vi "test Add Log File.vi"(8 "error in (no error)":errorcluster, 11 "TestCase in":refnum<class "Embedded Data Logger Scripting Unit Tests.lvclass">) -> (0 "error out":errorcluster, 3 "TestCase out":refnum<class "Embedded Data Logger Scripting Unit Tests.lvclass">)   [LabVIEW 2019, in "Embedded Data Logger Scripting Unit Tests.lvclass"]
uses:
  Embedded Data Logger Scripting Unit Tests.lvclass
  C:/Dev/GitHub/niveristand-custom-device-testing-tools/VeriStandScriptingTestCase/VeriStandScriptingTestCase.lvclass
  niveristand-custom-device-testing-tools/VeriStandScriptingTestCase/VeriStandScriptingTestCase.lvclass/VeriStandScriptingTestCase.ctl
  niveristand-custom-device-testing-tools/VeriStandScriptingTestCase/Read Target.vi
  NationalInstruments.VeriStand.SystemDefinitionAPI
  <vilib>/addons/_JKI Toolkits/VI Tester/TestCase.llb/TestCase.lvclass
  Embedded Data Logger Scripting.lvlib
  C:/Program Files (x86)/National Instruments/LabVIEW 2019/vi.lib/addons/_JKI Toolkits/VI Tester/TestCase.llb/TestCase.lvclass
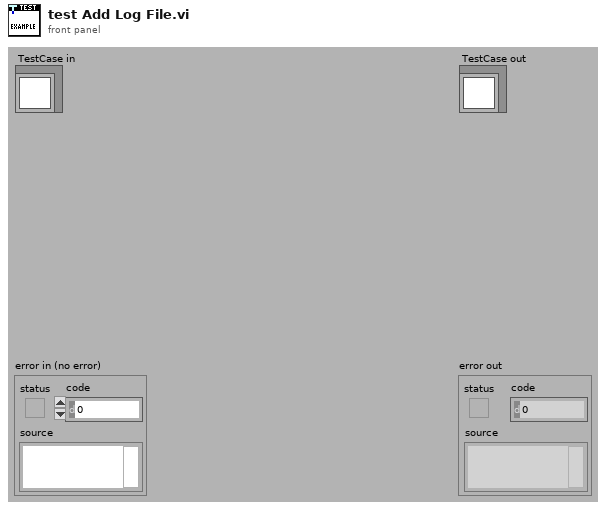
[diagram p1: front panel]
types:
  T1 = typedef "Custom Device API.lvlib/Custom Device Item Ref.ctl" = u64
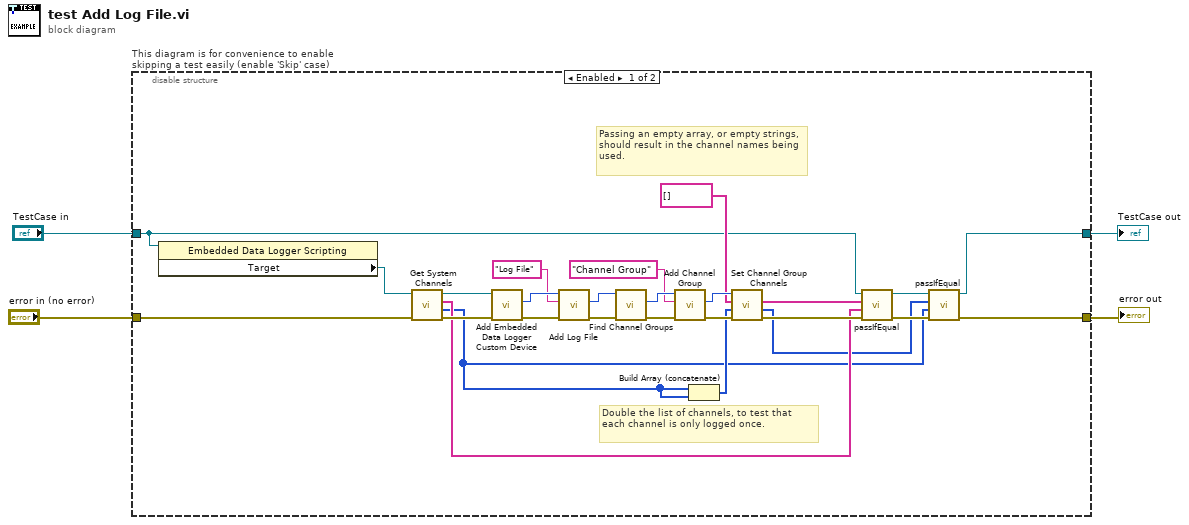
[diagram p0: block diagram]
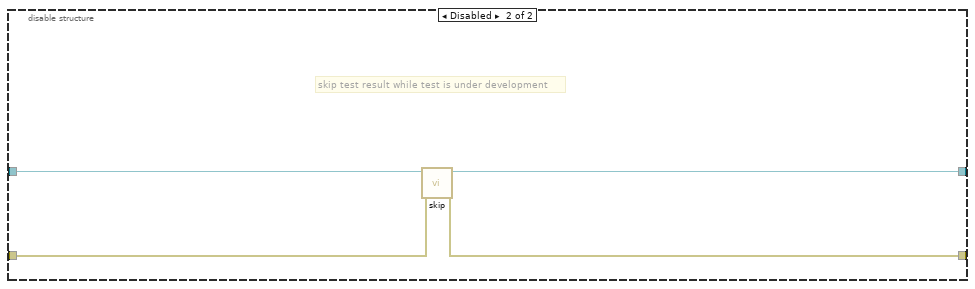
[diagram p2: hidden frame]
diagram:
  n1 = disable-structure "This diagram is for convenience to enable skipping a test easily (enable 'Skip' case)" shown="Enabled" {
    disable-tunnel: "TestCase in" -> [w13 w34]
    disable-tunnel: [w9 w32] -> w1
    disable-tunnel: [w8 w33] -> w3
    disable-tunnel: "error in (no error)" -> [w19 w31]
    frame Enabled {
      # "Passing an empty array, or empty strings, should result in the channel names being used."
      # "Double the list of channels, to test that each channel is only logged once."
      n2 = property class="Embedded Data Logger Scripting "(reference=w13) -> ("Target"=w22:refnum<k24>)  [unwired: 1 in, 2 out]
      n3 = call "Get System Channels.vi"("error in (no error)"=w19, "target in"=w22) -> ("error out"=w18:errorcluster, "channels"=w6:T1[], "names"=w11:string[], "target out"=w17:refnum<k24>)  [unwired: 6 in]
      n4 = call "Add Embedded Data Logger Custom Device.vi"("error in"=w18, "target in"=w17) -> ("error out"=w29:errorcluster, "embedded data logger"=w30:T1)  [unwired: 7 in, 1 out]
      n5 = call "Add Log File.vi"("error in"=w29, "log file name"="Log File", "embedded data logger in"=w30) -> ("error out"=w27:errorcluster, "log file"=w26:T1)  [unwired: 6 in, 1 out]
      n6 = call "Find Channel Groups.vi"("error in"=w27, "log file in"=w26) -> ("error out"=w25:errorcluster, "channel groups"=w24:T1)  [unwired: 7 in, 1 out]
      n7 = call "Add Channel Group.vi"("error in"=w25, "group name"="Channel Group", "channel groups in"=w24) -> ("error out"=w16:errorcluster, "channel group"=w21:T1)  [unwired: 6 in, 1 out]
      n8 = Build Array (concatenate)(w6, w6) -> (w15:T1[])
      n9 = call "Set Channel Group Channels.vi"("error in"=w16, "channels"=w15, "names"=string[] [], "channel group in"=w21) -> ("error out"=w14:errorcluster, "saved channels"=w5:T1[], "saved names"=w12:string[])  [unwired: 4 in, 1 out]
      n10 = call-dynamic "passIfEqual.vi"("error in (no error)"=w14, "y"=w11, "x"=w12, "TestCase in"=w13) -> ("error out"=w7:errorcluster, "TestCase out"=w10:refnum<class "Embedded Data Logger Scripting Unit Tests.lvclass">)  [unwired: 6 in]
      n11 = call-dynamic "passIfEqual.vi"("error in (no error)"=w7, "y"=w6, "x"=w5, "TestCase in"=w10) -> ("error out"=w8:errorcluster, "TestCase out"=w9:refnum<class "Embedded Data Logger Scripting Unit Tests.lvclass">)  [unwired: 6 in]
    }
    frame Disabled {
      # "skip test result while test is under development"
      n12 = call <vilib>:"skip.vi"("error in (no error)"=w31, "TestCase in"=w34) -> ("error out"=w33:errorcluster, "TestCase out"=w32:refnum<class "Embedded Data Logger Scripting Unit Tests.lvclass">)  [unwired: 8 in]
    }
  }
  "error out" <- w3
  "TestCase out" <- w1
